vi "formula.vi"   [LabVIEW 2014]
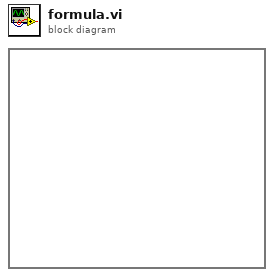
[diagram p0: block diagram]
diagram:
  n1 = formula code=""() -> ()
